vi "Rotate Flip Image.vi"(7 "Rotate?":bool, 10 "rect":T2={"left"=0, "top"=0, "right"=32, "bottom"=32}, 11 "Temp Icon In":picture) -> (2 "rect out":T1, 3 "Temp Icon Out":picture)   [LabVIEW 2017, in "lv_icon.lvlib"]
doc: "Rotate or Flip the glyph."
uses:
  <vilib>/LabVIEW Icon API/lv_icon/lv_icon.lvlib
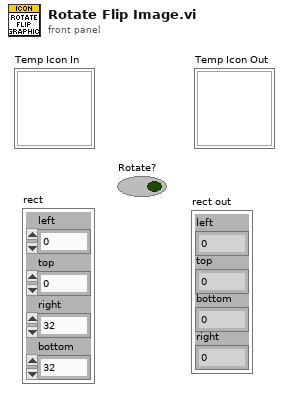
[diagram p1: front panel]
types:
  T1 = cluster{"left":i16, "top":i16, "bottom":i16, "right":i16}
  T2 = cluster{"left":i16, "top":i16, "right":i16, "bottom":i16}
  T3 = typedef "imagedata.ctl" = cluster{"image type":i32, "image depth":i32, "image":u8[], "mask":u8[], "colors":u32[], "Rectangle":cluster{"left":i16, "top":i16, "right":i16, "bottom":i16}}
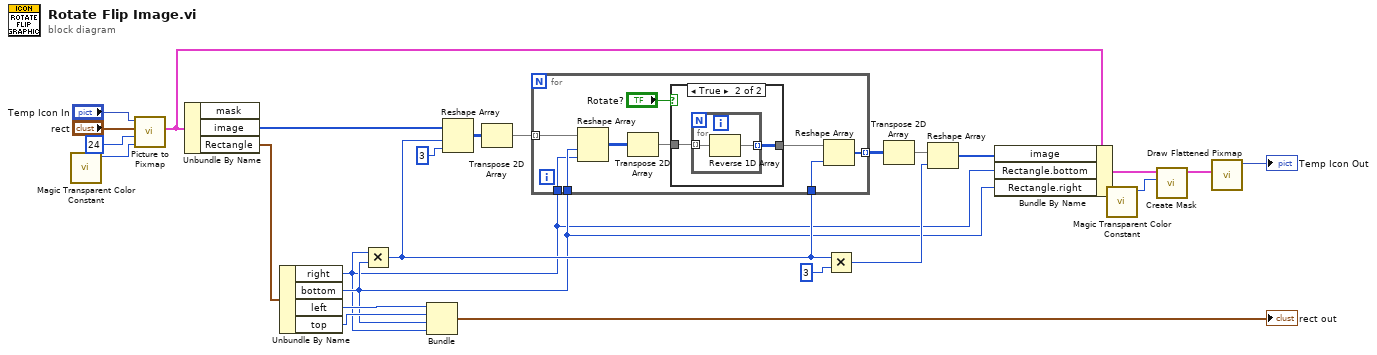
[diagram p0: block diagram]
diagram:
  n1 = call <vilib>:"Magic Transparent Color Constant.vi"() -> ("Magic transparent color constant"=w2:u32)  [unwired: 11 out]
  n2 = call <vilib>:"Picture to Pixmap.vi"("Background Color"=w2, "depth"=24, "rect"="rect", "picture"="Temp Icon In") -> ("image data"=w4:T3)  [unwired: 7 out]
  n3 = Unbundle By Name(w4) -> ("image"=w20:u8[], "Rectangle"=w13:T2)  [unwired: 1 out]
  n4 = Unbundle By Name(w13) -> ("right"=w5:i16, "bottom"=w6:i16, "left"=w8:i16, "top"=w7:i16)
  n5 = Multiply(x=w5, y=w6) -> (x*y=w19:i16)
  n6 = Bundle("left"=w8, "top"=w7, "bottom"=w6, "right"=w5) -> (→"rect out":T1)  [unwired: 1 out]
  n7 = Reshape Array(w20, w19, 3 ("dimension size")) -> (w24:u8[][])
  n8 = Transpose 2D Array(2D array=w24) -> (transposed array=w17:u8[][])
  n9 = for {
    tunnel: w17 -> [w34] mode=indexing
    tunnel: [w30] -> w16 mode=indexing
    tunnel: w5 -> [w31]
    tunnel: w6 -> [w32]
    tunnel: w19 -> [w33]
    n10 = Reshape Array(w34, w32, w31) -> (w28:u8[][])
    n11 = Transpose 2D Array(2D array=w28) -> (transposed array=w27:u8[][])
    n12 = case shown="True" "Rotate?" {
      tunnel: [w35 w36] -> w29
      tunnel: w27 -> [w35 w37]
      frame False {
      }
      frame True {
        n13 = for {
          tunnel: w37 -> [w39] mode=indexing
          tunnel: [w38] -> w36 mode=indexing
          n14 = Reverse 1D Array(array=w39) -> (reversed array=w38:u8[])
        }
      }
    }
    n15 = Reshape Array(w29, w33) -> (w30:u8[])
  }
  n16 = Multiply(x=w19, y=i16 3) -> (x*y=w21:i16)
  n17 = Transpose 2D Array(2D array=w16) -> (transposed array=w23:u8[][])
  n18 = Reshape Array(w23, w21) -> (w18:u8[])
  n19 = Bundle By Name(cluster=w4, "image"=w18, "Rectangle.bottom"=w5, "Rectangle.right"=w6) -> (w10:T3)
  n20 = call <vilib>:"Magic Transparent Color Constant.vi"() -> ("Magic transparent color constant"=w1:u32)  [unwired: 11 out]
  n21 = call <vilib>:"Create Mask.vi"("Mask Color (Black)"=w1, "image data"=w10) -> ("image data"=w9:T3)  [unwired: 2 in, 7 out]
  n22 = call <vilib>:"Draw Flattened Pixmap.vi"("image data"=w9) -> ("new picture"=→"Temp Icon Out":picture)  [unwired: 1 in, 7 out]
